vi "UnregisterEvents.vi"(8 "Error In":errorcluster, 10 "Root Actor's Enqueuer":refnum<class "Message Enqueuer.lvclass">, 11 "Nested Actor's EnqueuerArray":refnum<class "Message Enqueuer.lvclass">[](array[class])) -> (0 "Error Out":errorcluster)   [LabVIEW 2019, in "TestBench.lvlib" / "TestBench.lvclass"]
uses:
  TestBench.lvclass
  <vilib>/ActorFramework/Message Enqueuer/Message Enqueuer.lvclass
  <vilib>/NI/Event Source Actor/Event Source/Event Source Messages/Unregister Msg/Unregister Msg.lvclass/Unregister Msg.ctl
  <vilib>/ActorFramework/Message Enqueuer/Message Enqueuer.lvclass/Message Enqueuer.ctl
  <vilib>/ActorFramework/Message Enqueuer/Enqueue.vi
  <vilib>/NI/Event Source Actor/Event Source/Event Source Messages/Unregister Msg/Unregister Msg.lvclass
  C:/Program Files (x86)/National Instruments/LabVIEW 2019/vi.lib/ActorFramework/Message/Message.lvclass
  <vilib>/ActorFramework/Message Priority Queue/Priority Enqueue.vi
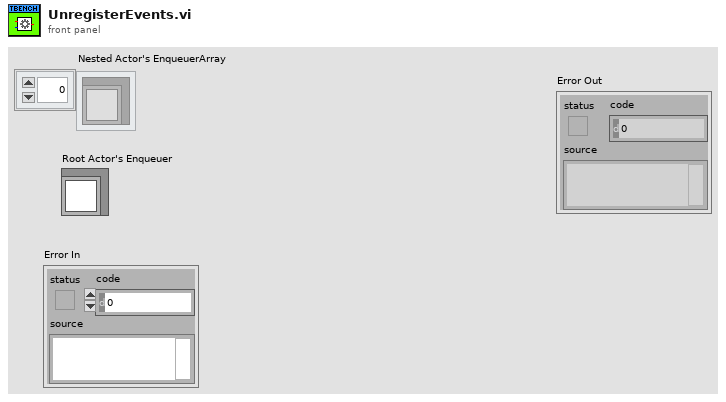
[diagram p1: front panel]
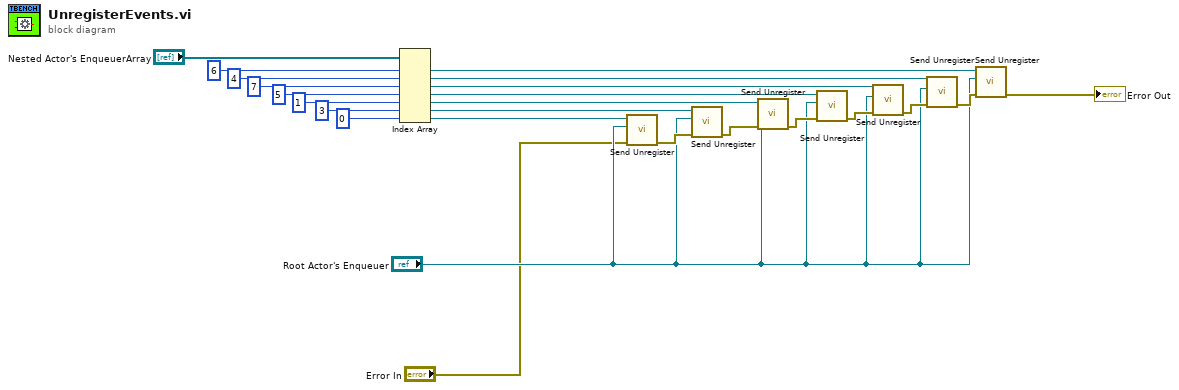
[diagram p0: block diagram]
diagram:
  n1 = Index Array(array="Nested Actor's EnqueuerArray", index #1=6 ("index"), index #2=4 ("index"), index #3=7 ("index"), index #4=5 ("index"), index #5=1 ("index"), index #6=3 ("index"), index #7=0 ("index")) -> (element #1=w18:refnum<class "Message Enqueuer.lvclass">, element #2=w14:refnum<class "Message Enqueuer.lvclass">, element #3=w15:refnum<class "Message Enqueuer.lvclass">, element #4=w16:refnum<class "Message Enqueuer.lvclass">, element #5=w17:refnum<class "Message Enqueuer.lvclass">, element #6=w3:refnum<class "Message Enqueuer.lvclass">, element #7=w2:refnum<class "Message Enqueuer.lvclass">)
  n2 = call <vilib>:"Send Unregister.vi"("Error In"="Error In", "Registrant Address"="Root Actor's Enqueuer", "Event Source Address"=w2) -> ("Error Out"=w8:errorcluster)  [unwired: 7 in, 1 out]
  n3 = call <vilib>:"Send Unregister.vi"("Error In"=w8, "Registrant Address"="Root Actor's Enqueuer", "Event Source Address"=w3) -> ("Error Out"=w6:errorcluster)  [unwired: 7 in, 1 out]
  n4 = call <vilib>:"Send Unregister.vi"("Error In"=w6, "Registrant Address"="Root Actor's Enqueuer", "Event Source Address"=w17) -> ("Error Out"=w13:errorcluster)  [unwired: 7 in, 1 out]
  n5 = call <vilib>:"Send Unregister.vi"("Error In"=w13, "Registrant Address"="Root Actor's Enqueuer", "Event Source Address"=w16) -> ("Error Out"=w12:errorcluster)  [unwired: 7 in, 1 out]
  n6 = call <vilib>:"Send Unregister.vi"("Error In"=w12, "Registrant Address"="Root Actor's Enqueuer", "Event Source Address"=w15) -> ("Error Out"=w11:errorcluster)  [unwired: 7 in, 1 out]
  n7 = call <vilib>:"Send Unregister.vi"("Error In"=w11, "Registrant Address"="Root Actor's Enqueuer", "Event Source Address"=w14) -> ("Error Out"=w10:errorcluster)  [unwired: 7 in, 1 out]
  n8 = call <vilib>:"Send Unregister.vi"("Error In"=w10, "Registrant Address"="Root Actor's Enqueuer", "Event Source Address"=w18) -> ("Error Out"=→"Error Out":errorcluster)  [unwired: 7 in, 1 out]
